vi "Eliminar TDMS.vi"(8 "error in":errorcluster, 10 "semaphore":T1) -> (0 "error out":errorcluster, 2 "semaphore out":T1)   [LabVIEW 2015]
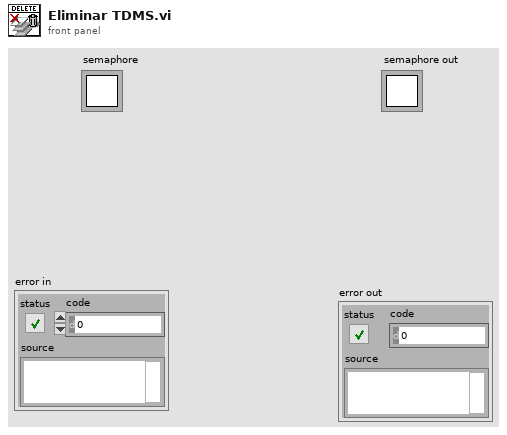
[diagram p1: front panel]
types:
  T1 = typedef "Semaphore RefNum" = refnum<k1>
  T2 = enum16{"open", "open or create", "create or replace", "create", "open (read-only)"}
  T3 = cluster{"tdms control out":refnum<k34>, "tdms historial out":refnum<k34>, "tdms sinc out":refnum<k34>}
  T4 = cluster{"tdms file out":refnum<k34>, "tdms file out":refnum<k34>, "tdms file out":refnum<k34>}
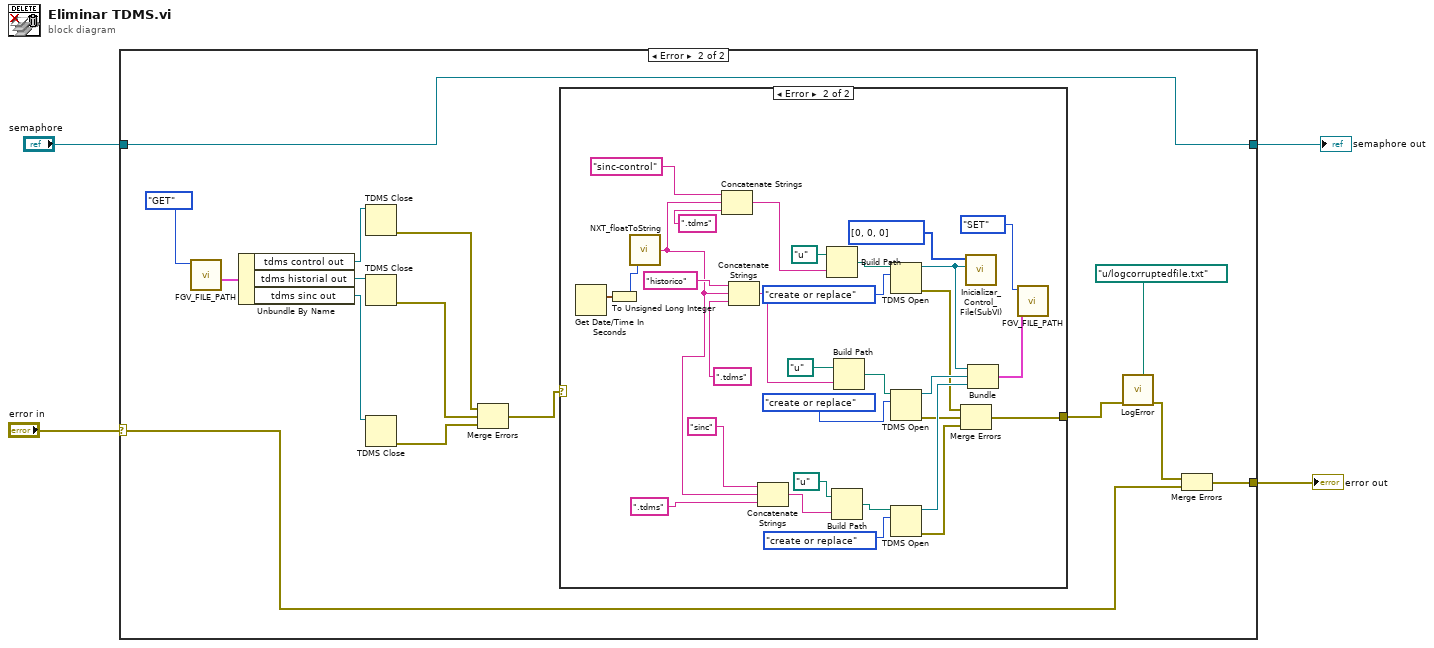
[diagram p0: block diagram]
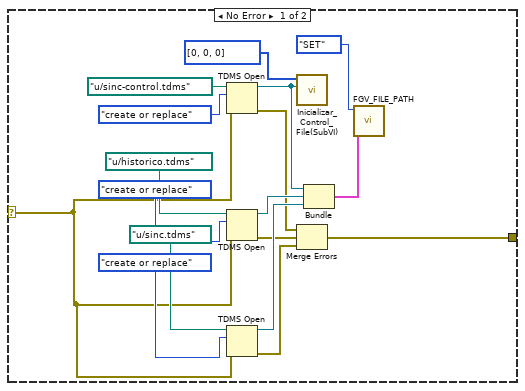
[diagram p3: hidden frame]
diagram:
  n1 = case shown="Error" "error in" {
    selector: "error in" -> [w5 w16]
    tunnel: [w6 w10] -> w3
    tunnel: "semaphore" -> [w6 w10]
    tunnel: [w5 w15] -> w1
    frame No Error {
    }
    frame Error {
      n2 = call "FGV_FILE_PATH.vi"("Function"=enum16{"GET", "SET"}."GET") -> ("Data Out"=w20:T3)  [unwired: 10 in]
      n3 = Unbundle By Name(w20) -> ("tdms control out"=w19:refnum<k34>, "tdms historial out"=w18:refnum<k34>, "tdms sinc out"=w17:refnum<k34>)
      n4 = TDMS Close(11:w19) -> (0:w9:errorcluster)  [unwired: 1 in, 1 out]
      n5 = TDMS Close(11:w18) -> (0:w8:errorcluster)  [unwired: 1 in, 1 out]
      n6 = TDMS Close(11:w17) -> (0:w7:errorcluster)  [unwired: 1 in, 1 out]
      n7 = Merge Errors(w9, w8, w7) -> (w11:errorcluster)
      n8 = case shown="Error" w11 {
        selector: w11 -> [w22 _]
        tunnel: [w23 w57] -> w14
        frame No Error {
          n9 = TDMS Open(8:w22, 10:T2."create or replace" ("operation (0:open)"), 11:path "u:/sinc-control.tdms" ("file path")) -> (0:w26:errorcluster, 3:w35:refnum<k34>)  [unwired: 4 in]
          n10 = TDMS Open(8:w22, 10:T2."create or replace" ("operation (0:open)"), 11:path "u:/historico.tdms" ("file path")) -> (0:w25:errorcluster, 3:w33:refnum<k34>)  [unwired: 4 in]
          n11 = TDMS Open(8:w22, 10:T2."create or replace" ("operation (0:open)"), 11:path "u:/sinc.tdms" ("file path")) -> (0:w24:errorcluster, 3:w29:refnum<k34>)  [unwired: 4 in]
          n12 = call "Inicializar_Control_File(SubVI).vi"("tdms file"=w35, "Offsets"=i64[] [0, 0, 0]) -> ()  [unwired: 9 in, 1 out]
          n13 = Merge Errors(w26, w25, w24) -> (w23:errorcluster)
          n14 = Bundle("tdms file out"=w35, "tdms file out"=w33, "tdms file out"=w29) -> (w28:T4)  [unwired: 1 in]
          n15 = call "FGV_FILE_PATH.vi"("Data In"=w28, "Function"=enum16{"GET", "SET"}."SET") -> ()  [unwired: 9 in, 1 out]
        }
        frame Error {
          n16 = Get Date/Time In Seconds() -> (seconds since 1Jan1904=w50:timestamp)
          n17 = To Unsigned Long Integer(number=w50) -> (unsigned 32bit integer=w51:u32)
          n18 = call <vilib>:"NXT_floatToString.vi"("number"=w51) -> ("string"=w41:string)
          n19 = Concatenate Strings("sinc-control" ("remote path"), w41, ".tdms" ("string")) -> (w39:string)
          n20 = Concatenate Strings("historico" ("remote path"), w41, ".tdms" ("string")) -> (w46:string)
          n21 = Concatenate Strings("sinc" ("remote path"), w41, ".tdms" ("string")) -> (w44:string)
          n22 = Build Path(base path=path "u:/", name or relative path=w39) -> (appended path=w56:path)
          n23 = Build Path(base path=path "u:/", name or relative path=w44) -> (appended path=w54:path)
          n24 = Build Path(base path=path "u:/", name or relative path=w46) -> (appended path=w55:path)
          n25 = TDMS Open(10:T2."create or replace" ("operation (0:open)"), 11:w56) -> (0:w60:errorcluster, 3:w67:refnum<k34>)  [unwired: 5 in]
          n26 = TDMS Open(10:T2."create or replace" ("operation (0:open)"), 11:w55) -> (0:w59:errorcluster, 3:w66:refnum<k34>)  [unwired: 5 in]
          n27 = TDMS Open(10:T2."create or replace" ("operation (0:open)"), 11:w54) -> (0:w58:errorcluster, 3:w63:refnum<k34>)  [unwired: 5 in]
          n28 = Merge Errors(w60, w59, w58) -> (w57:errorcluster)
          n29 = call "Inicializar_Control_File(SubVI).vi"("tdms file"=w67, "Offsets"=i64[] [0, 0, 0]) -> ()  [unwired: 9 in, 1 out]
          n30 = Bundle("tdms file out"=w67, "tdms file out"=w66, "tdms file out"=w63) -> (w62:T4)  [unwired: 1 in]
          n31 = call "FGV_FILE_PATH.vi"("Data In"=w62, "Function"=enum16{"GET", "SET"}."SET") -> ()  [unwired: 9 in, 1 out]
        }
      }
      n32 = call "LogError.vi"("Error In"=w14, "Path"=path "u:/logcorruptedfile.txt") -> ("Error Out"=w13:errorcluster)  [unwired: 8 in, 1 out]
      n33 = Merge Errors(w13, w16) -> (w15:errorcluster)
    }
  }
  "error out" <- w1
  "semaphore out" <- w3
